vi "Add Resource (Decimation).vi"(0 "instance":u8, 1 "harness type":T1, 2 "acq in":refnum<class "niUSRP Rx DSP v2 FPGA.lvclass">, 3 "collection builder in":refnum<class "Collection Builder.lvclass">, 5 "IP enabled":bool, 7 "overclock":refnum<k21>, 9 "overclock factor":u8, 12 "channel":u8) -> (13 "acq out":refnum<class "niUSRP Rx DSP v2 FPGA.lvclass">, 14 "collection builder out":refnum<class "Collection Builder.lvclass">)   [LabVIEW 2025, in "niUSRP Rx DSP v2 FPGA.lvclass"]
uses:
  niUSRP Rx DSP v2 FPGA.lvclass
  <instrlib>/_niInstr/Instruction Framework/v1/FPGA/Collection Builder/Collection Builder.lvclass
  <instrlib>/_niInstr/DSP Control/Common/v2/FPGA/Resampling/Harness Type.ctl
  <instrlib>/_niInstr/DSP Control/Interface/v1/FPGA/Decimation/IQ 18-bit/Decimation Interface (IQ 18-bit).lvclass
  <instrlib>/_niInstr/Instruction Framework/v1/FPGA/Helper Classes/Single Address Space Collection/Single Address Space Collection.lvclass
  C:/Program Files/NI/LVAddons/niidl/1/instr.lib/_niInstr/Instruction Framework/v1/FPGA/Interfaces/Address Space Collection/Address Space Collection.lvclass
  <instrlib>/_niInstr/DSP Control/Common/v2/FPGA/Decimation/IQ 18-bit Frac/Fractional Decimator (IQ 18-bit).lvclass
  C:/Program Files/NI/LVAddons/niidl/1/instr.lib/_niInstr/DSP Control/Interface/v1/FPGA/Decimation/IQ 18-bit/Decimation Interface (IQ 18-bit).lvclass
  <instrlib>/_niInstr/DSP Control/Common/v2/FPGA/Decimation/IQ 18-bit HB/Halfband Decimator (IQ 18-bit).lvclass
  <instrlib>/_niInstr/Basic Elements/v1/FPGA/niInstr Basic Elements v1 FPGA.lvlib
  <instrlib>/_niInstr/DSP Control/Common/v2/FPGA/Resampling/Resampler Harness.lvclass
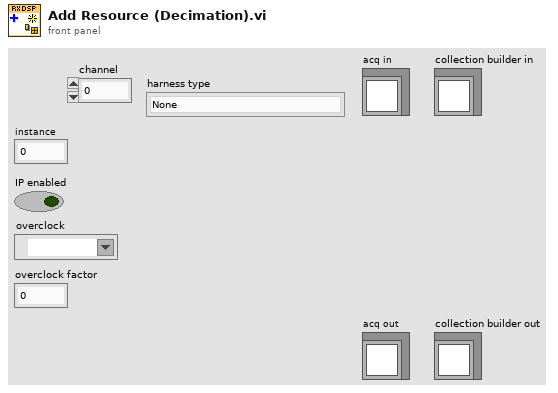
[diagram p1: front panel]
types:
  T1 = typedef "niInstr DSP Control Common v2 FPGA.lvlib/Resampler Harness.lvclass/Harness Type.ctl" = enum16{"None", "Integer Linear", "Integer List", "Integer-Exponential", "Fixed Rational", "Fractional (16-bit Delay)", "Fractional (18-bit Delay)", "Rational List", "External", "External and Fractional"}
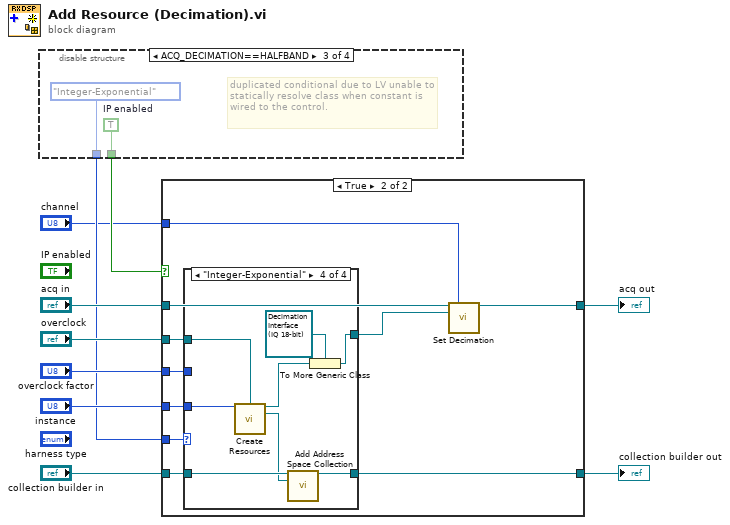
[diagram p0: block diagram]
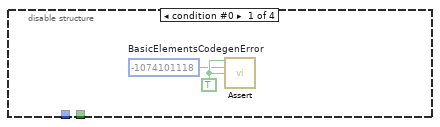
[diagram p2: hidden frame]
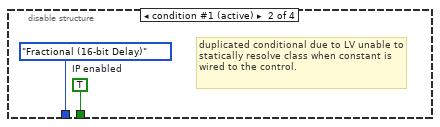
[diagram p3: hidden frame]
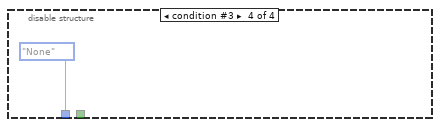
[diagram p4: hidden frame]
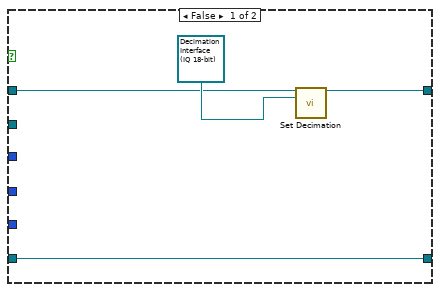
[diagram p5: hidden frame]
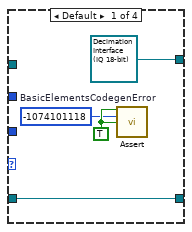
[diagram p6: hidden frame]
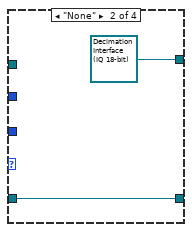
[diagram p7: hidden frame]
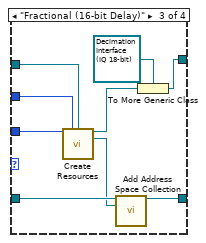
[diagram p8: hidden frame]
diagram:
  n1 = disable-structure shown="ACQ_DECIMATION==HALFBAND" {
    disable-tunnel: [_ w14 w16 _] -> w3
    disable-tunnel: [_ Harness_Type."Fractional (16-bit Delay)" ("harness type") Harness_Type."Integer-Exponential" ("harness type") Harness_Type."None" ("harness type")] -> w2
    frame condition #0 {
      w12 = TRUE ("assert")
      w11 = -1074101118  # BasicElementsCodegenError
      n2 = call <instrlib>:"Assert.vi"("assert"=w12, "error code"=w11, "enable show error"=w12) -> ()  [unwired: 13 in]
    }
    frame condition #1 (active) {
      w14 = TRUE  # IP enabled
      # "duplicated conditional due to LV unable to statically resolve class when constant is wired to the control."
    }
    frame condition #2 {
      w16 = TRUE  # IP enabled
      # "duplicated conditional due to LV unable to statically resolve class when constant is wired to the control."
    }
    frame condition #3 {
    }
  }
  n3 = case shown="True" w3 {
    tunnel: "collection builder in" -> [w21 w24]
    tunnel: [w21 w23] -> w9
    tunnel: "instance" -> [_ w31]
    tunnel: "acq in" -> [w18 w27]
    tunnel: [w20 w26] -> w6
    tunnel: w2 -> [_ w30]
    tunnel: "overclock" -> [_ w29]
    tunnel: "overclock factor" -> [_ w28]
    tunnel: "channel" -> [_ w22]
    frame False {
      n4 = call-dynamic "Set Decimation.vi"("acq in"=w18, "decimation"=refnum<class "Decimation Interface (IQ 18-bit).lvclass"> refnum ("iq impairments")) -> ("acq out"=w20:refnum<class "niUSRP Rx DSP v2 FPGA.lvclass">)  [unwired: 13 in]
    }
    frame True {
      n5 = case shown="\"Integer-Exponential\"" w30 {
        tunnel: w31 -> [_ _ w46 w54]
        tunnel: w29 -> [_ _ w45 w53]
        tunnel: w28 -> [_ _ w44 _]
        tunnel: [refnum<class "Decimation Interface (IQ 18-bit).lvclass"> refnum ("decimation") refnum<class "Decimation Interface (IQ 18-bit).lvclass"> refnum ("decimation") w41 w50] -> w25
        tunnel: w24 -> [w32 w36 w40 w49]
        tunnel: [w32 w36 w38 w47] -> w23
        frame Default {
          w35 = TRUE ("assert")
          w34 = -1074101118  # BasicElementsCodegenError
          n6 = call <instrlib>:"Assert.vi"("assert"=w35, "error code"=w34, "enable show error"=w35) -> ()  [unwired: 13 in]
        }
        frame "None" {
        }
        frame "Fractional (16-bit Delay)" {
          n7 = call <instrlib>:"Create Resources.vi"("instance"=w46, "overclock factor"=w44, "overclock"=w45) -> ("decimation"=w42:refnum<class "Fractional Decimator (IQ 18-bit).lvclass">, "decimation registers"=w39:refnum<class "Single Address Space Collection.lvclass">)  [unwired: 11 in]
          n8 = call <instrlib>:"Add Address Space Collection.vi"("collection builder in"=w40, "address space collection"=w39) -> ("collection builder out"=w38:refnum<class "Collection Builder.lvclass">)  [unwired: 13 in]
          n9 = To More Generic Class(target class=refnum<class "Decimation Interface (IQ 18-bit).lvclass"> refnum ("decimation"), reference=w42) -> (generic class reference=w41:refnum<class "Decimation Interface (IQ 18-bit).lvclass">)
        }
        frame "Integer-Exponential" {
          n10 = call <instrlib>:"Create Resources.vi"("instance"=w54, "overclock"=w53) -> ("decimation"=w51:refnum<class "Halfband Decimator (IQ 18-bit).lvclass">, "decimation registers"=w48:refnum<class "Single Address Space Collection.lvclass">)  [unwired: 12 in]
          n11 = call <instrlib>:"Add Address Space Collection.vi"("collection builder in"=w49, "address space collection"=w48) -> ("collection builder out"=w47:refnum<class "Collection Builder.lvclass">)  [unwired: 13 in]
          n12 = To More Generic Class(target class=refnum<class "Decimation Interface (IQ 18-bit).lvclass"> refnum ("decimation"), reference=w51) -> (generic class reference=w50:refnum<class "Decimation Interface (IQ 18-bit).lvclass">)
        }
      }
      n13 = call-dynamic "Set Decimation.vi"("acq in"=w27, "channel"=w22, "decimation"=w25) -> ("acq out"=w26:refnum<class "niUSRP Rx DSP v2 FPGA.lvclass">)  [unwired: 12 in]
    }
  }
  "collection builder out" <- w9
  "acq out" <- w6
